vi "SysInfo-SubWCRev.vi"(11 "path":path) -> (0 "error out":errorcluster, 2 "HasModifications":bool, 3 "Revision":i32)   [LabVIEW 2020]
uses:
  <vilib>/regexp/Match Regular Expression.xnode
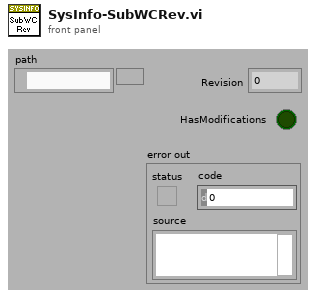
[diagram p1: front panel]
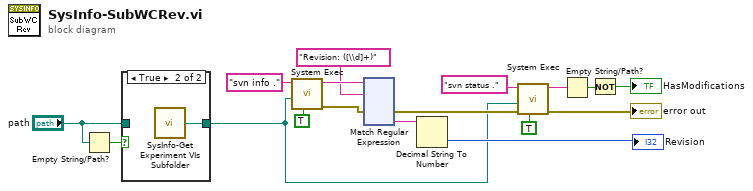
[diagram p0: block diagram]
diagram:
  n1 = Empty String/Path?(string/path="path") -> (empty?=w2:bool)
  n2 = case shown="True" w2 {
    tunnel: [w18 w19] -> w5
    tunnel: "path" -> [w18 _]
    frame False {
    }
    frame True {
      n3 = call "SysInfo-Get Experiment VIs Subfolder.vi"() -> ("full path"=w19:path)  [unwired: 5 in]
    }
  }
  n4 = call <vilib>:"System Exec.vi"("run minimized? (F)"=TRUE, "working directory"=w5, "command line"="svn info .") -> ("error out"=w10:errorcluster, "standard output"=w13:string)  [unwired: 5 in, 2 out]
  n5 = xnode "Match Regular Expression"("input string"=w13, "regular expression"="Revision: ([\\d]+)", "error in"=w10) -> ("error out"=w8:errorcluster, "submatch 1"=w11:string)  [unwired: 3 in, 4 out]
  n6 = Decimal String To Number(string=w11) -> (number=→"Revision":i32)  [unwired: 2 in, 1 out]
  n7 = call <vilib>:"System Exec.vi"("run minimized? (F)"=TRUE, "error in (no error)"=w8, "working directory"=w5, "command line"="svn status .") -> ("error out"=→"error out":errorcluster, "standard output"=w7:string)  [unwired: 4 in, 2 out]
  n8 = Empty String/Path?(string/path=w7) -> (empty?=w6:bool)
  n9 = Not(x=w6) -> (.not. x?=→"HasModifications":bool)
